vi "Main.vi"() -> ()   [LabVIEW 2014]
uses:
  EMC API/EMC_Typedef_Motor_Parameters.ctl
  Typedef/Typedef_Motor_Action.ctl
  FPGA_VI/SubVIs/Pulse Trigger.ctl
  Functional_Global/Typedef_FPGA_Interface_Action.ctl
  <vilib>/Motion/Express/_s/nimc.ex.clearFaults.clearFaults.axis.vi
  <vilib>/Motion/Express/_s/nimc.ex.power.power.axis.vi
  <vilib>/Motion/Express/_s/nimc.ex.resetPosition.resetPosition.axis.vi
  <vilib>/Utility/error.llb/Error Cluster From Error Code.vi
  <vilib>/rvi/errors/niLvFpgaAdjustHostInterfaceError.vi
  <vilib>/Motion/Express/_s/nimc.ex.read.readTrajectoryData.axis.vi
  <vilib>/Motion/Express/_s/nimc.ex.read.readMotionIO.axis.vi
  <vilib>/Motion/Express/_s/nimc.ex.findReferenceMove.startReferenceMove.axis.modeReverseLimit.vi
  <vilib>/Motion/Express/_s/nimc.ex.findReferenceMove.startReferenceMove.axis.modeHome.vi
  <vilib>/Motion/Express/_s/nimc.ex.findReferenceMove.startReferenceMove.axis.modeForwardLimit.vi
  <vilib>/Motion/BlockNode/FB.NIMotion.xnode
  <vilib>/rvi/interface/nirviReadWriteControl/nirviReadWriteControl.xnode
  NiFpgaLv.dll
  <vilib>/rvi/interface/Simulation/niFpgaSimulationCallBeginRW.vi
panel:
  out "Axis Positions 2":fxp<+/-,64,32>[](array[numeric])
  out "TPeriod (ticks)":u32
  in  "TPulse (ticks)":i32=2000
  in  "Ta (ticks)":i32
  in  "Tb (ticks)":i32
  in  "Number of pulses (N)":i32=4
  out "Remainder (ticks)":i32
  out "Processed Pulse":i32[](array[numeric])
  out "Ta Error":bool
  out "Tb Error":bool
  out "Tpulse Error":bool
  in  "Process Engine Mode":enum16{"Auto Calc Tpulse", "Auto Calc Tb"}(ring)
  in  "Reset?":bool
  in  "Clear FIFO":bool
  in  "TDelay (ticks)":i32
  out "Process Engine State":T1
  out "Armed":bool
  in  "Axis 5 Mode":enum16{"No Sync", "Sync with Sensor"}(ring)
  out "Time elapsed (ticks)":u32
  out "Toggle Iterations":u32
  in  "Sensor Sync DIR":bool
  out "FIFO Read Timed Out?":bool
  in  "Mark Sensor Simulation":bool
  out "FIFO Write Timed Out?":bool
  out "FIFO Elements to Read":u32
  in  "Use sim?":bool=TRUE
  out "Mod3/DIO0":bool
  in  "Home 5":bool
  in  "Home 4":bool
  in  "Home 3":bool
  in  "Home 2":bool
  in  "Home 1":bool
  in  "velocity":dbl=1000.0
  in  "Positions":dbl[](array[numeric])=[5000.0, 5000.0, 5000.0, 5000.0, 5000.0]
  in  "resource":refnum<k21>="Axis 1"
  out "HOME active":bool
  out "REV active":bool
  out "FWD active":bool
  out "XY Graph":cluster{"X Array":dbl[], "Y Array":dbl[]}(graph)
  in  "interval":dbl=0.01 format="%#_13g"
  in  "Gear in/out":enum16{"Gear in", "Gear out"}(ring)
  in  "denominator":i32=1
  in  "numerator":i32=1
  in  "Master Axis":T2(ring)
  out "Array":dbl[](array[knob]) scale=0.0..1600.0
  in  "Clear Errors":bool
  in  "Command":T3
  in  "Motion Parameters":T4={"position"=1000.0, "velocity"=1000.0, "acceleration"=10000.0, "deceleration"=10000.0, "accel. jerk"=10000.0, "decel. jerk"=10000.0}
  in  "Axis Index":T2(ring)
  out "error":errorcluster
  out "Numeric":i32=519
  in  "Stop all motors":bool
  in  "Execute Command":bool
  in  "stop":bool
  out "Axis Velocities":T5(graph)
  out "Axis Positions":T5(graph)
  # "Coordinate Move"
  # "Mark Sensor Sync Options"
  # "FIFO Check"
  # "Limit Switch Status"
  # "Ta + (TPulse * 2 * N) + Tb = TPeriod"
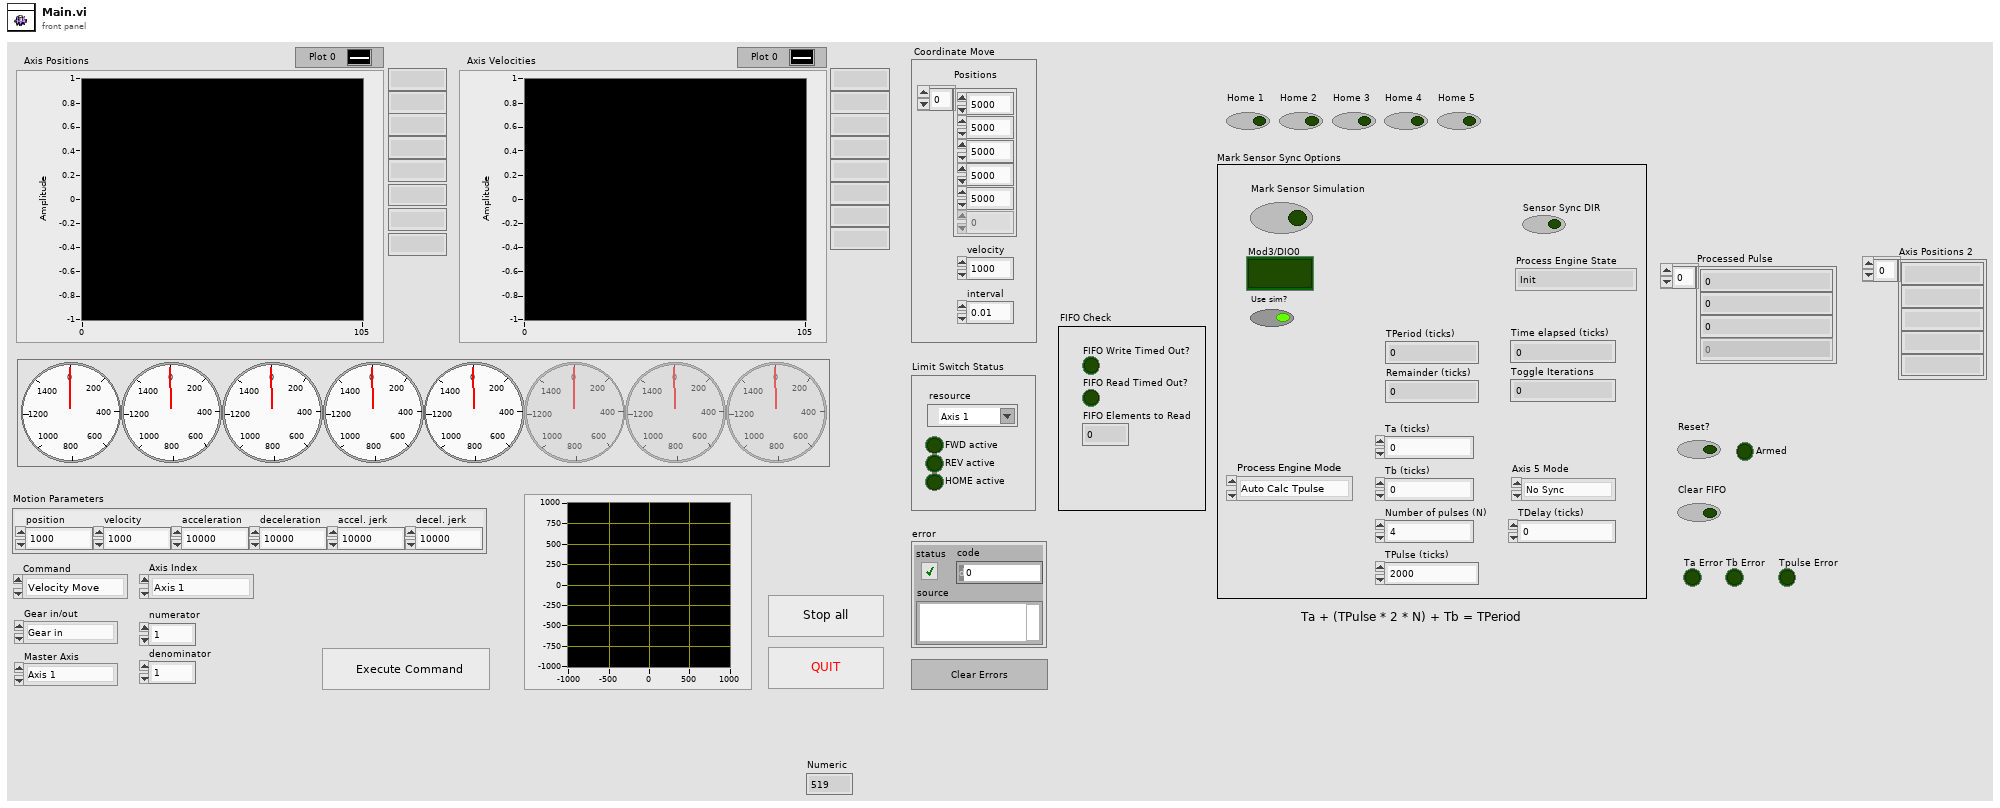
[diagram p1: front panel]
types:
  T1 = typedef "Pulse Trigger.ctl" = enum16{"Init", "Armed", "Processing"}
  T2 = enum16{"Axis 1", "Axis 2", "Axis 3", "Axis 4", "Axis 5", "Axis 6", "Axis 7", "Axis 8"}
  T3 = typedef "Typedef_Motor_Action.ctl" = enum16{"Velocity Move", "REL Pos Move", "ABS Pos Move", "Stop", "Reset Position", "Coordinate_move", "Contour_move", "Gearing", "Find Fwd Limit", "Find Rev Limit", "Find Home"}
  T4 = typedef "EMC_Typedef_Motor_Parameters.ctl" = cluster{"position":dbl, "velocity":dbl, "acceleration":dbl, "deceleration":dbl, "accel. jerk":dbl, "decel. jerk":dbl}
  T5 = cluster{"[0]":dbl, "[1]":dbl, "[2]":dbl, "[3]":dbl, "[4]":dbl, "[5]":dbl, "[6]":dbl, "[7]":dbl}
  T6 = typedef "Typedef_FPGA_Interface_Action.ctl" = enum16{"Initialize FPGA", "Get FPGA Reference", "Close FPGA"}
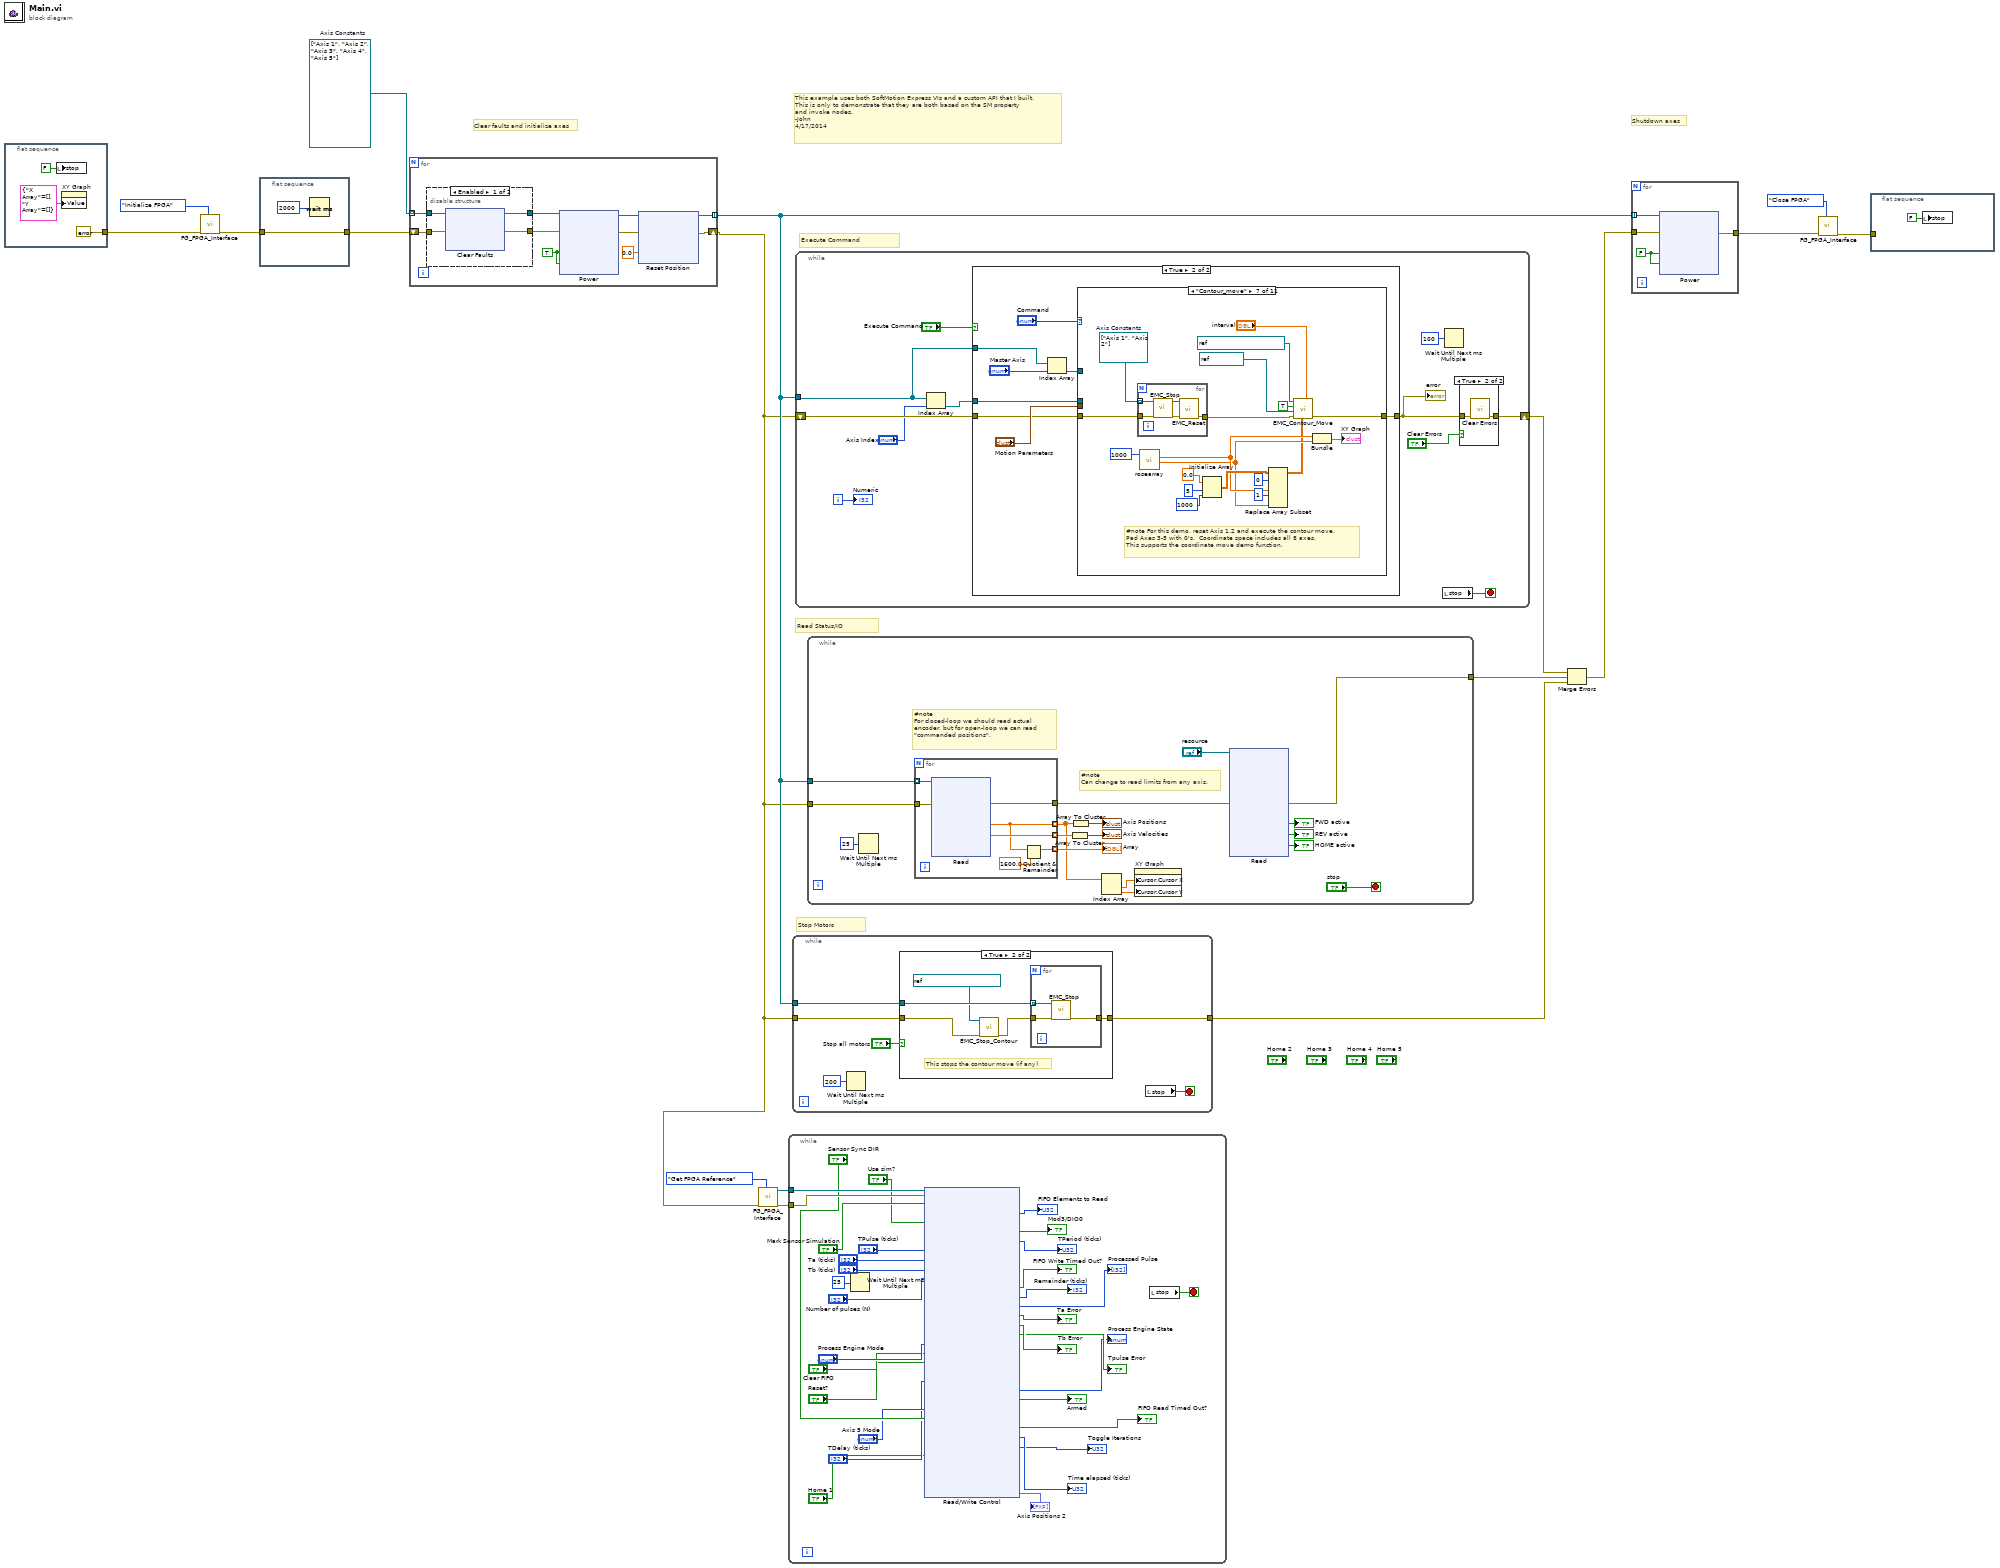
[diagram p0: block diagram]
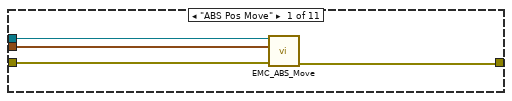
[diagram p6: hidden frame]
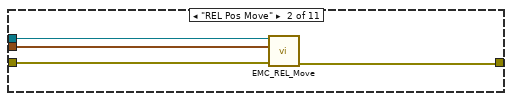
[diagram p7: hidden frame]
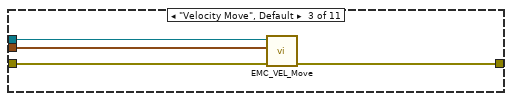
[diagram p8: hidden frame]
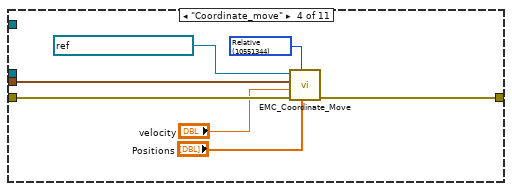
[diagram p9: hidden frame]
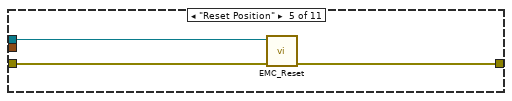
[diagram p10: hidden frame]
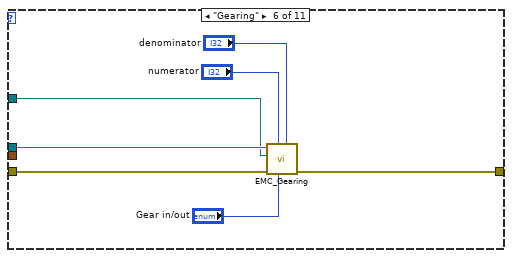
[diagram p11: hidden frame]
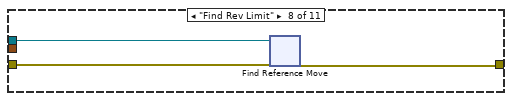
[diagram p12: hidden frame]
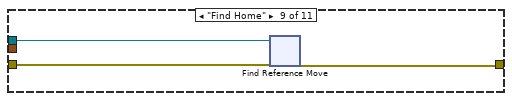
[diagram p13: hidden frame]
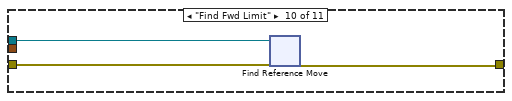
[diagram p14: hidden frame]
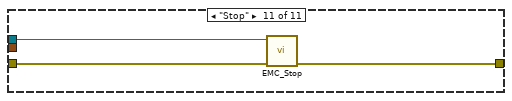
[diagram p15: hidden frame]
diagram:
  w16 = refnum<k21>[] ["Axis 1", "Axis 2", "Axis 3", "Axis 4", "Axis 5"]  # Axis Constants
  # "Clear faults and initialize axes"
  # "This example uses both SoftMotion Express VIs and a custom API that I built.\nThis is only to demonstrate that they are both based on the SM property\nand invoke nodes. \n-John\n4/17/2014"
  # "Shutdown axes"
  # "Execute Command"
  # "Read Status/IO"
  # "Stop Motors"
  n1 = flat-sequence {
    tunnel: [errorcluster {"status"=FALSE, "code"=0, "source"=""} ("error in (no error)")] -> w13
    frame #0 {
      n2 = local write "stop"(FALSE ("stop")) -> ()
      n3 = property on="XY Graph" class="XYGraph (strict)"("Value"=cluster{"X Array":dbl[], "Y Array":dbl[]} {"X Array"=[], "Y Array"=[]} ("XY Graph")) -> ()  [unwired: 2 in, 2 out]
    }
  }
  n4 = call "FG_FPGA_Interface.vi"("Action"=Typedef_FPGA_Interface_Action."Initialize FPGA", "error in"=w13) -> ("error out"=w3:errorcluster)  [unwired: 8 in, 1 out]
  n5 = flat-sequence {
    tunnel: w3 -> [w21]
    tunnel: [w21] -> w2
    frame #0 {
      n6 = Wait (ms)(milliseconds to wait=u32 2000) -> ()  [unwired: 1 out]
    }
  }
  n7 = for {
    tunnel: w16 -> [w27] mode=indexing
    tunnel: [w28] -> w9 mode=indexing
    shift-right: [w23] -> w1
    shift-left: w2 -> [w24]
    w32 = TRUE ("enable axis")
    n8 = disable-structure shown="Enabled" {
      disable-tunnel: w27 -> [w36 w42]
      disable-tunnel: [w35 w42] -> w26
      disable-tunnel: [w34 w41] -> w25
      disable-tunnel: w24 -> [w33 _]
      frame Enabled {
        n9 = xnode ("Clear Faults")("resource"=w36, "error in"=w33) -> ("resource out"=w35:refnum<k21>, "error out"=w34:errorcluster)
      }
      frame Disabled {
      }
    }
    n10 = xnode ("Power")("enable axis"=w32, "enable drive"=w32, "resource"=w26, "error in"=w25) -> ("resource out"=w31:refnum<k21>, "error out"=w30:errorcluster)
    n11 = xnode ("Reset Position")("position"=0.0, "resource"=w31, "error in"=w30) -> ("resource out"=w28:refnum<k21>, "error out"=w23:errorcluster)
  }
  n12 = call "FG_FPGA_Interface.vi"("Action"=Typedef_FPGA_Interface_Action."Get FPGA Reference", "error in"=w1) -> ("error out"=w5:errorcluster, "FPGA VI Reference Out"=w4:refnum<k20>)  [unwired: 8 in]
  n13 = while {
    tunnel: w5 -> [w86]
    tunnel: w4 -> [w87]
    stop <- w89 stop-if-true
    n14 = Wait Until Next ms Multiple(millisecond multiple=u32 25) -> ()  [unwired: 1 out]
    n15 = xnode "Read/Write Control"("FPGA VI Reference In"=w87, "error in"=w86, "Mark Sensor Simulation"="Mark Sensor Simulation", "Use sim?"="Use sim?", "TPulse (ticks)"="TPulse (ticks)", "Ta (ticks)"="Ta (ticks)", "Tb (ticks)"="Tb (ticks)", "Number of pulses (N)"="Number of pulses (N)", "Process Engine Mode"="Process Engine Mode", "Reset?"="Reset?", "Clear FIFO"="Clear FIFO", "TDelay (ticks)"="TDelay (ticks)", "Axis 5 Mode"="Axis 5 Mode", "Sensor Sync DIR"="Sensor Sync DIR", "Home 1"="Home 1") -> ("FIFO Elements to Read"=→"FIFO Elements to Read":u32, "Mod3/DIO0"=→"Mod3/DIO0":bool, "TPeriod (ticks)"=→"TPeriod (ticks)":u32, "FIFO Write Timed Out?"=→"FIFO Write Timed Out?":bool, "Remainder (ticks)"=→"Remainder (ticks)":i32, "Processed Pulse"=→"Processed Pulse":i32[], "Ta Error"=→"Ta Error":bool, "Tb Error"=→"Tb Error":bool, "Tpulse Error"=→"Tpulse Error":bool, "Process Engine State"=→"Process Engine State":enum16{"Init", "Armed", "Processing"}, "Armed"=→"Armed":bool, "FIFO Read Timed Out?"=→"FIFO Read Timed Out?":bool, "Time elapsed (ticks)"=→"Time elapsed (ticks)":u32, "Toggle Iterations"=→"Toggle Iterations":u32, "Axis Positions"=→"Axis Positions 2":fxp<+/-,64,32>[])  [unwired: 6 out]
    n16 = local read "stop"() -> (w89:bool)
  }
  n17 = while {
    tunnel: w1 -> [w94]
    tunnel: w9 -> [w92]
    tunnel: [w90] -> w17
    stop <- w95 stop-if-true
    n18 = Wait Until Next ms Multiple(millisecond multiple=u32 200) -> ()  [unwired: 1 out]
    n19 = case shown="True" "Stop all motors" {
      tunnel: w94 -> [w96 w99]
      tunnel: [w96 w101] -> w90
      tunnel: w92 -> [_ w100]
      frame False {
      }
      frame True {
        # "This stops the contour move (if any)"
        n20 = call "EMC_Stop_Contour.vi"("error in (no error)"=w99, "coordinate"=refnum<k21> "Coordinate Space 1") -> ("error out"=w97:errorcluster)  [unwired: 9 in]
        n21 = for {
          tunnel: w97 -> [w104]
          tunnel: w100 -> [w102] mode=indexing
          tunnel: [w103] -> w101
          n22 = call "EMC_Stop.vi"("error in (no error)"=w104, "axis"=w102) -> ("error out"=w103:errorcluster)  [unwired: 8 in, 1 out]
        }
      }
    }
    n23 = local read "stop"() -> (w95:bool)
  }
  n24 = while {
    tunnel: w9 -> [w106]
    shift-right: [w107] -> w12
    shift-left: w1 -> [w111]
    i -> [w115]
    stop <- w105 stop-if-true
    n25 = Index Array(array=w106, index="Axis Index") -> (element=w112:refnum<k21>)
    n26 = case shown="True" "Execute Command" {
      tunnel: w111 -> [w119 w126]
      tunnel: w112 -> [_ w125]
      tunnel: [w119 w124] -> w108
      tunnel: w106 -> [_ w121]
      frame False {
      }
      frame True {
        n27 = Index Array(array=w121, index="Master Axis") -> (element=w120:refnum<k21>)
        n28 = case shown="\"Contour_move\"" "Command" {
          tunnel: "Motion Parameters" -> [w128 w132 w139 w140 _ _ _ _ _ _ _]
          tunnel: w126 -> [w131 w135 w138 w146 w149 w156 w168 w182 w201 w222 w242]
          tunnel: w125 -> [w129 w133 w137 _ w148 w155 _ w181 w200 w221 w240]
          tunnel: [w130 w134 w136 w145 w147 w154 w175 w183 w202 w223 w241] -> w124
          tunnel: w120 -> [_ _ _ _ _ w150 _ _ _ _ _]
          frame "ABS Pos Move" {
            n29 = call "EMC_ABS_Move.vi"("error in (no error)"=w131, "Motion Parameters"=w128, "axis"=w129) -> ("error out"=w130:errorcluster)  [unwired: 8 in]
          }
          frame "REL Pos Move" {
            n30 = call "EMC_REL_Move.vi"("error in (no error)"=w135, "Motion Parameters"=w132, "axis"=w133) -> ("error out"=w134:errorcluster)  [unwired: 8 in]
          }
          frame "Velocity Move", Default {
            n31 = call "EMC_VEL_Move.vi"("error in (no error)"=w138, "Motion Parameters"=w139, "axis"=w137) -> ("error out"=w136:errorcluster)  [unwired: 8 in]
          }
          frame "Coordinate_move" {
            w143 = 10551344 items=["Relative"=10551344, "Absolute"=10551337, "Relative To Capture"=10551345, "Velocity"=10551346, "Polyline"=11600101] ("line move mode")
            n32 = call "EMC_Coordinate_Move.vi"("position[]"="Positions", "line move mode"=w143, "error in (no error)"=w146, "velocity"="velocity", "Motion Parameters"=w140, "resource"=refnum<k21> "Coordinate Space 1") -> ("error out"=w145:errorcluster)  [unwired: 5 in]
          }
          frame "Reset Position" {
            n33 = call "EMC_Reset.vi"("error in (no error)"=w149, "axis"=w148) -> ("error out"=w147:errorcluster)  [unwired: 9 in]
          }
          frame "Gearing" {
            n34 = call "EMC_Gearing.vi"("denominator"="denominator", "Gear in/out"="Gear in/out", "numerator"="numerator", "error in (no error)"=w156, "master axis"=w150, "axis"=w155) -> ("error out"=w154:errorcluster)  [unwired: 5 in]
          }
          frame "Contour_move" {
            w166 = refnum<k21>[] ["Axis 1", "Axis 2"]  # Axis Constants
            # "#note For this demo, reset Axis 1,2 and execute the contour move.\nPad Axes 3-5 with 0's.  Coordinate space includes all 8 axes.\nThis supports the coordinate move demo function."
            n35 = for {
              tunnel: w168 -> [w179]
              tunnel: [w180] -> w167
              tunnel: w166 -> [w177] mode=indexing
              n36 = call "EMC_Stop.vi"("error in (no error)"=w179, "axis"=w177) -> ("error out"=w178:errorcluster, "axis out"=w176:refnum<k21>)  [unwired: 8 in]
              n37 = call "EMC_Reset.vi"("error in (no error)"=w178, "axis"=w176) -> ("error out"=w180:errorcluster)  [unwired: 9 in]
            }
            n38 = call "rosearray.vi"("Iterations"=u32 1000) -> ("Y Array"=w158:dbl[], "X Array"=w159:dbl[])  [unwired: 5 in, 1 out]
            n39 = Initialize Array(0.0 ("element"), 5 ("dimension size"), 1000 ("dimension size")) -> (w163:dbl[][])
            n40 = Replace Array Subset(array=w163, new element #1=w159, index (row) #1=0 ("index (row)"), new element #2=w158, index (row) #2=1 ("index (row)")) -> (w157:dbl[][])  [unwired: 2 in]
            n41 = call "EMC_Contour_Move.vi"("interval"="interval", "points[][]"=w157, "error in (no error)"=w167, "table"=refnum<k21> "Table 1" ("resource"), "overwrite"=TRUE, "coordinate"=refnum<k21> "Coordinate Space 1" ("resource")) -> ("error out"=w175:errorcluster)  [unwired: 5 in]
            n42 = Bundle("X Array"=w159, "Y Array"=w158) -> (→"XY Graph":cluster{"X Array":dbl[], "Y Array":dbl[]})  [unwired: 1 in]
          }
          frame "Find Rev Limit" {
            n43 = xnode "Find Reference Move"("resource"=w181, "error in"=w182) -> ("error out"=w183:errorcluster)  [unwired: 9 in, 2 out]
          }
          frame "Find Home" {
            n44 = xnode "Find Reference Move"("resource"=w200, "error in"=w201) -> ("error out"=w202:errorcluster)  [unwired: 11 in, 2 out]
          }
          frame "Find Fwd Limit" {
            n45 = xnode "Find Reference Move"("resource"=w221, "error in"=w222) -> ("error out"=w223:errorcluster)  [unwired: 9 in, 2 out]
          }
          frame "Stop" {
            n46 = call "EMC_Stop.vi"("error in (no error)"=w242, "axis"=w240) -> ("error out"=w241:errorcluster)  [unwired: 8 in, 1 out]
          }
        }
      }
    }
    "error" <- w108
    n47 = local read "stop"() -> (w105:bool)
    n48 = Wait Until Next ms Multiple(millisecond multiple=u32 100) -> ()  [unwired: 1 out]
    n49 = case shown="True" "Clear Errors" {
      tunnel: w108 -> [w116 w118]
      tunnel: [w116 w117] -> w107
      frame False {
      }
      frame True {
        n50 = call <vilib>:"Clear Errors.vi"("error in (no error)"=w118) -> ("error out"=w117:errorcluster)  [unwired: 5 in, 1 out]
      }
    }
    "Numeric" <- w115
  }
  n51 = while {
    tunnel: w1 -> [w256]
    tunnel: w9 -> [w255]
    tunnel: [w244] -> w15
    stop <- "stop" stop-if-true
    # "#note \nCan change to read limits from any axis."
    # "#note \nFor closed-loop we should read actual \nencoder, but for open-loop we can read\n\"commanded positions\"."
    n52 = Wait Until Next ms Multiple(millisecond multiple=u32 25) -> ()  [unwired: 1 out]
    n53 = for {
      tunnel: [w294] -> w246
      tunnel: [w289] -> w253 mode=indexing
      tunnel: [w293] -> w259 mode=indexing
      tunnel: w256 -> [w292]
      tunnel: w255 -> [w291] mode=indexing
      tunnel: [w288] -> w254 mode=indexing
      n54 = xnode ("Read")("resource"=w291, "error in"=w292) -> ("commanded position"=w289:dbl, "commanded vel."=w293:dbl, "error out"=w294:errorcluster)  [unwired: 2 out]
      n55 = Quotient & Remainder(x=w289, y=1600.0) -> (x-y*floor(x/y)=w288:dbl)  [unwired: 1 out]
    }
    "Array" <- w254
    n56 = Array To Cluster(array=w259) -> (cluster=→"Axis Velocities":T5)
    n57 = Array To Cluster(array=w253) -> (cluster=→"Axis Positions":T5)
    n58 = Index Array(array=w253) -> (element #1=w252:dbl, element #2=w251:dbl)  [unwired: 2 in]
    n59 = property on="XY Graph" class="XYGraph (strict)"("Cursor.Cursor X"=w252, "Cursor.Cursor Y"=w251) -> ()  [unwired: 2 in, 2 out]
    n60 = xnode ("Read")("resource"="resource", "error in"=w246) -> ("fwd. limit active"=→"FWD active":bool, "rev. limit active"=→"REV active":bool, "home active"=→"HOME active":bool, "error out"=w244:errorcluster)  [unwired: 6 out]
  }
  n61 = Merge Errors(w12, w15, w17) -> (w10:errorcluster)
  n62 = for {
    tunnel: w9 -> [w305] mode=indexing
    tunnel: [w303] -> w11
    tunnel: w10 -> [w302]
    w304 = FALSE ("enable axis")
    n63 = xnode ("Power")("enable axis"=w304, "enable drive"=w304, "resource"=w305, "error in"=w302) -> ("error out"=w303:errorcluster)  [unwired: 1 out]
  }
  n64 = call "FG_FPGA_Interface.vi"("Action"=Typedef_FPGA_Interface_Action."Close FPGA", "error in"=w11) -> ("error out"=w14:errorcluster)  [unwired: 8 in, 1 out]
  n65 = flat-sequence {
    tunnel: w14 -> [_]
    frame #0 {
      n66 = local write "stop"(FALSE ("stop")) -> ()
    }
  }
